vi "Set Value.vi"(8 "Error In":errorcluster, 10 "Value":dbl, 11 "Number Widget In":refnum<class "Number Widget.lvclass">) -> (0 "Error Out":errorcluster, 3 "Number Widget Out":refnum<class "Number Widget.lvclass">)   [LabVIEW 2014, in "6. Reusing Components Dynamically.lvlib" / "Number Widget.lvclass"]
doc: "Sets the value of the LCD and slider.\n\n\nCopyright (c) 2019 Sze Howe Koh.\nThis code is licensed under the MIT license."
uses:
  Number Widget.lvclass
  Number Widget.lvclass/Number Widget.ctl
  <vilib>/addons/LQ/Qwt/QwtAbstractSlider/QwtAbstractSlider.lvclass
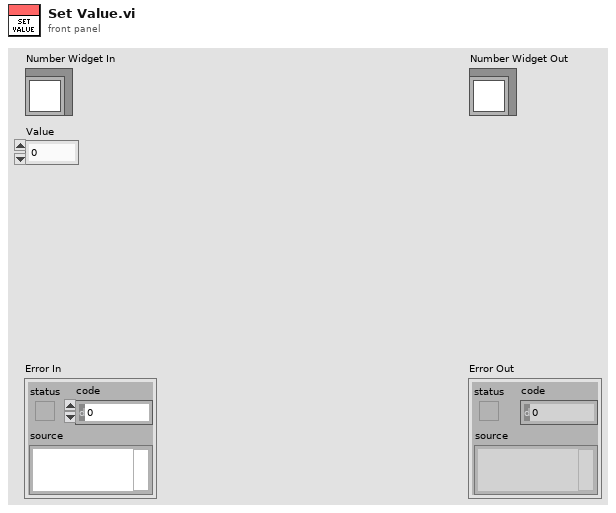
[diagram p1: front panel]
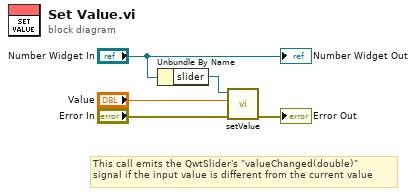
[diagram p0: block diagram]
diagram:
  # "This call emits the QwtSlider's \"valueChanged(double)\"\nsignal if the input value is different from the current value"
  n1 = Unbundle By Name("Number Widget In") -> ("slider"=w3:refnum<class "QwtSlider.lvclass">)
  n2 = call <vilib>:"setValue.vi"("Error In"="Error In", "val"="Value", "QwtAbstractSlider In"=w3) -> ("Error Out"=→"Error Out":errorcluster)  [unwired: 7 in, 1 out]
  "Number Widget Out" <- "Number Widget In"
